vi "调节电压.vi"(4 "电压减少":bool, 6 "电压增加":bool, 8 "错误输入（无错误）":errorcluster, 9 "电压调节速度":u16(ring) items=["1", "2", "3"], 10 "通道 2":u16(ring) items=["V1", "V2"], 11 "引用":refnum<visa-resource-name>) -> (5 "引用输出":refnum<visa-resource-name>, 7 "错误输出":errorcluster)   [LabVIEW 2018]
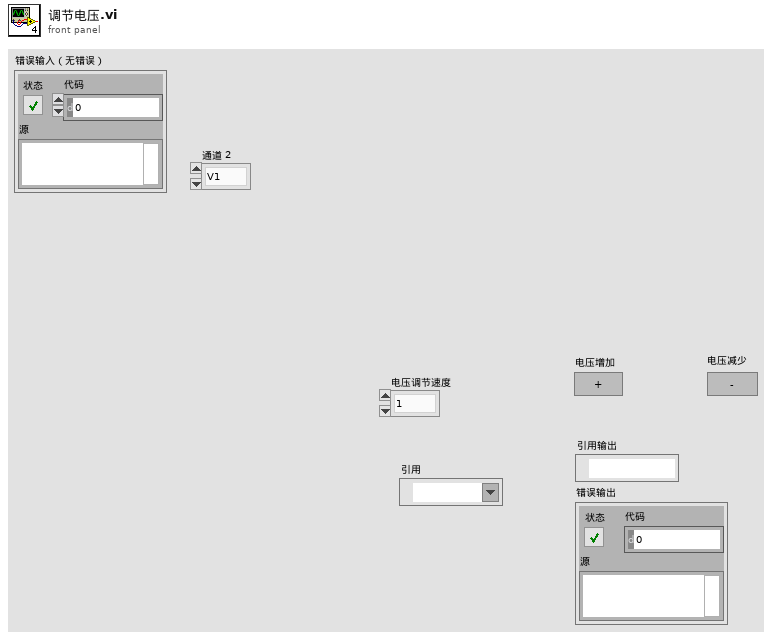
[diagram p1: front panel]
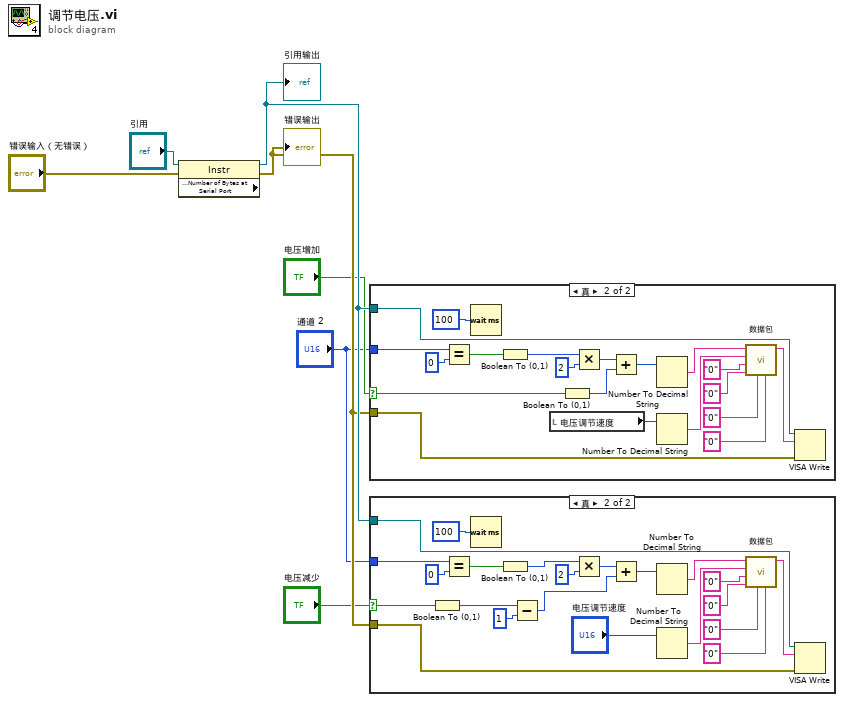
[diagram p0: block diagram]
diagram:
  n1 = property class="Instr" props=["Serial Settings:Number of Bytes at Serial Port"](reference="引用", error in="错误输入（无错误）") -> (reference out=w7:refnum<visa-resource-name>, error out=w6:errorcluster)  [unwired: 1 out]
  "引用输出" <- w7
  "错误输出" <- w6
  n2 = case shown="真" "电压增加" {
    selector: "电压增加" -> [_ w21]
    tunnel: w7 -> [_ w10]
    tunnel: w6 -> [_ w9]
    tunnel: "通道 2" -> [_ w8]
    frame False {
    }
    frame True {
      n3 = Equal?(x=w8, y=0) -> (x = y?=w25:bool)
      n4 = Wait (ms)(milliseconds to wait=100) -> ()  [unwired: 1 out]
      n5 = Boolean To (0,1)(Boolean=w25) -> (0, 1=w24:i16)
      n6 = local read "电压调节速度"() -> (w18:u16)
      n7 = Boolean To (0,1)(Boolean=w21) -> (0, 1=w20:i16)
      n8 = Multiply(x=w24, y=2) -> (x*y=w22:i32)
      n9 = Add(x=w22, y=w20) -> (x+y=w19:i32)
      n10 = Number To Decimal String(number=w19) -> (decimal integer string=w17:string)  [unwired: 1 in]
      n11 = Number To Decimal String(number=w18) -> (decimal integer string=w16:string)  [unwired: 1 in]
      n12 = call "数据包.vi"("字符串 6"="0", "字符串 5"="0", "字符串 4"="0", "字符串 3"="0", "字符串 2"=w16, "字符串1"=w17) -> ("连接的字符串"=w12:string)  [unwired: 5 in]
      n13 = VISA Write(VISA resource name=w10, write buffer=w12, error in (no error)=w9) -> ()  [unwired: 3 out]
    }
  }
  n14 = case shown="真" "电压减少" {
    selector: "电压减少" -> [_ w42]
    tunnel: w7 -> [_ w30]
    tunnel: w6 -> [_ w29]
    tunnel: "通道 2" -> [_ w28]
    frame False {
    }
    frame True {
      n15 = Boolean To (0,1)(Boolean=w42) -> (0, 1=w43:i16)
      n16 = Equal?(x=w28, y=0) -> (x = y?=w47:bool)
      n17 = Wait (ms)(milliseconds to wait=100) -> ()  [unwired: 1 out]
      n18 = Boolean To (0,1)(Boolean=w47) -> (0, 1=w46:i16)
      n19 = Subtract(x=w43, y=1) -> (x-y=w40:i32)
      n20 = Multiply(x=w46, y=2) -> (x*y=w44:i32)
      n21 = Add(x=w44, y=w40) -> (x+y=w39:i32)
      n22 = Number To Decimal String(number=w39) -> (decimal integer string=w38:string)  [unwired: 1 in]
      n23 = Number To Decimal String(number="电压调节速度") -> (decimal integer string=w35:string)  [unwired: 1 in]
      n24 = call "数据包.vi"("字符串 6"="0", "字符串 5"="0", "字符串 4"="0", "字符串 3"="0", "字符串 2"=w35, "字符串1"=w38) -> ("连接的字符串"=w37:string)  [unwired: 5 in]
      n25 = VISA Write(VISA resource name=w30, write buffer=w37, error in (no error)=w29) -> ()  [unwired: 3 out]
    }
  }
